vi "DAQ Relay States - Filter Out.vi"(0 "TSM Context":T1, 5 "RLY in":string[](array[string]), 11 "error in (no error)":errorcluster, 12 "State":bool) -> (4 "Relay Filtered out":string[](array[string]), 15 "error out":errorcluster)   [LabVIEW 2019]
uses:
  <vilib>/NI_TestStand_SemiconductorModule/NI_TestStand_Semiconductor_Module.lvlibp/PinMap/General/SemiconductorModuleContext.ctl
  <vilib>/NI_TestStand_SemiconductorModule/NI_TestStand_Semiconductor_Module.lvlibp/1abvi3w/instr.lib/niSwitch/niswitch.llb/niSwitch Relay Action.ctl
  <vilib>/NI_TestStand_SemiconductorModule/NI_TestStand_Semiconductor_Module.lvlibp
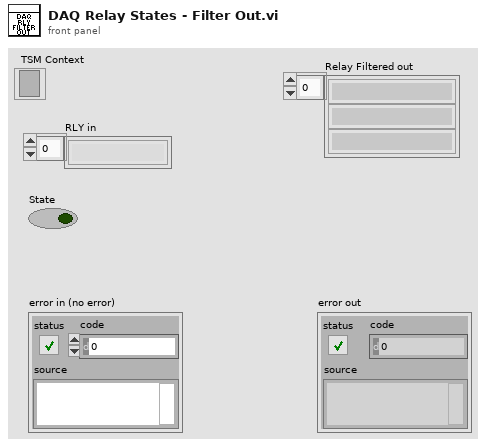
[diagram p1: front panel]
types:
  T1 = typedef "NI_TestStand_Semiconductor_Module.lvlibp/SemiconductorModuleContext.ctl" = refnum<k7>
  T2 = typedef "NI_TestStand_Semiconductor_Module.lvlibp/niSwitch Relay Action.ctl" = i32
  T3 = typedef "DAQ Relay Pins.ctl" = cluster{"DAQ Relay":tag, "Relay Action":T2}
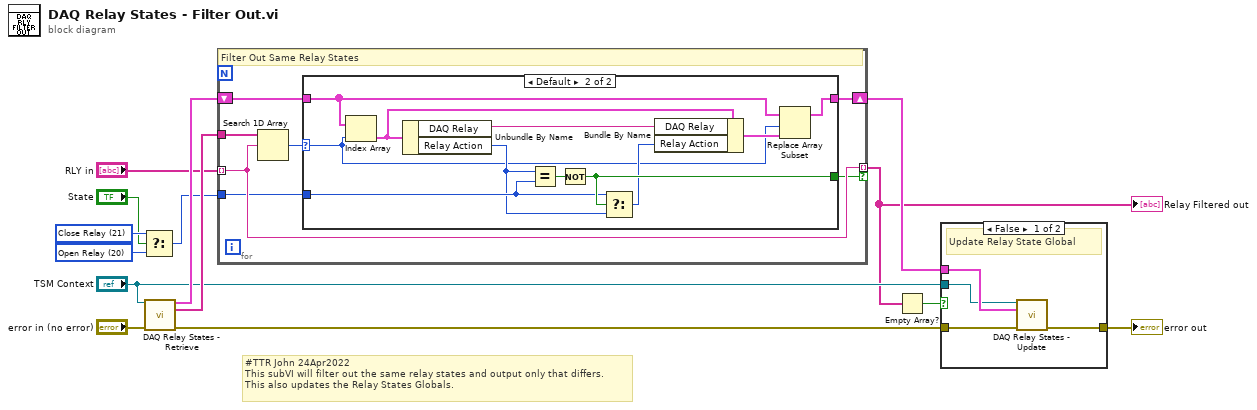
[diagram p0: block diagram]
diagram:
  w4 = T2 20 items=["Open Relay"=20, "Close Relay"=21] ("Relay Action")
  w3 = T2 21 items=["Open Relay"=20, "Close Relay"=21] ("Relay Action")
  # "#TTR John 24Apr2022\nThis subVI will filter out the same relay states and output only that differs.\nThis also updates the Relay States Globals."
  n1 = Select(t=w3, s="State", f=w4) -> (s? t:f=w2:T2)
  n2 = call "DAQ Relay States - Retrieve.vi"("TSM Context"="TSM Context", "error in (no error)"="error in (no error)") -> ("DAQ States - Out"=w14:T3[], "DAQ Relay Names String"=w13:string[], "error out"=w9:errorcluster)  [unwired: 11 in]
  n3 = for {
    tunnel: w13 -> [w21]
    tunnel: "RLY in" -> [w20] mode=indexing
    tunnel: w2 -> [w18]
    tunnel: [w20] -> w6 mode=indexing if=w19
    shift-right: [w16] -> w10
    shift-left: w14 -> [w17]
    # "Filter Out Same Relay States"
    n4 = Search 1D Array(1D array=w21, element=w20) -> (index of element=w15:i32)  [unwired: 1 in]
    n5 = case shown="Default" w15 {
      selector: w15 -> [_ w23]
      tunnel: [_ w30] -> w19
      tunnel: w18 -> [_ w29]
      tunnel: w17 -> [w22 w26]
      tunnel: [w22 w24] -> w16
      frame -1 {
      }
      frame Default {
        n6 = Index Array(array=w26, index=w23) -> (element=w32:T3)
        n7 = Unbundle By Name(w32) -> ("DAQ Relay"=w31:tag, "Relay Action"=w28:T2)
        n8 = Equal?(x=w28, y=w29) -> (x = y?=w33:bool)
        n9 = Not(x=w33) -> (.not. x?=w30:bool)
        n10 = Select(t=w29, s=w30, f=w28) -> (s? t:f=w27:T2)
        n11 = Bundle By Name(cluster=w32, "DAQ Relay"=w31, "Relay Action"=w27) -> (w25:T3)
        n12 = Replace Array Subset(array=w26, new element=w25, index=w23) -> (w24:T3[])
      }
    }
  }
  "Relay Filtered out" <- w6
  n13 = Empty Array?(array=w6) -> (empty?=w5:bool)
  n14 = case shown="False" w5 {
    tunnel: w10 -> [w37 _]
    tunnel: w9 -> [w36 w38]
    tunnel: [w35 w38] -> w8
    tunnel: "TSM Context" -> [w34 _]
    frame False {
      # "Update Relay State Global"
      n15 = call "DAQ Relay States - Update.vi"("TSM Context"=w34, "DAQ States - Out"=w37, "error in (no error)"=w36) -> ("error out"=w35:errorcluster)  [unwired: 12 in]
    }
    frame True {
      # "Skip Update if Empty"
    }
  }
  "error out" <- w8
